vi "AnaliseOffline.vi"() -> ()   [LabVIEW 2014, in "Aquisicao de Dados.lvlib"]
uses:
  Aquisicao de Dados.lvlib
panel:
  in  "Amostras de Gravação":i32=100
  out "Waveform Graph":waveform(dbl)[](graph)
  in  "Método de Entrada":T1(ring)
  in  "Amostras por Iteração":i32=2000
  in  "Error In":errorcluster
  out "Error Out":errorcluster
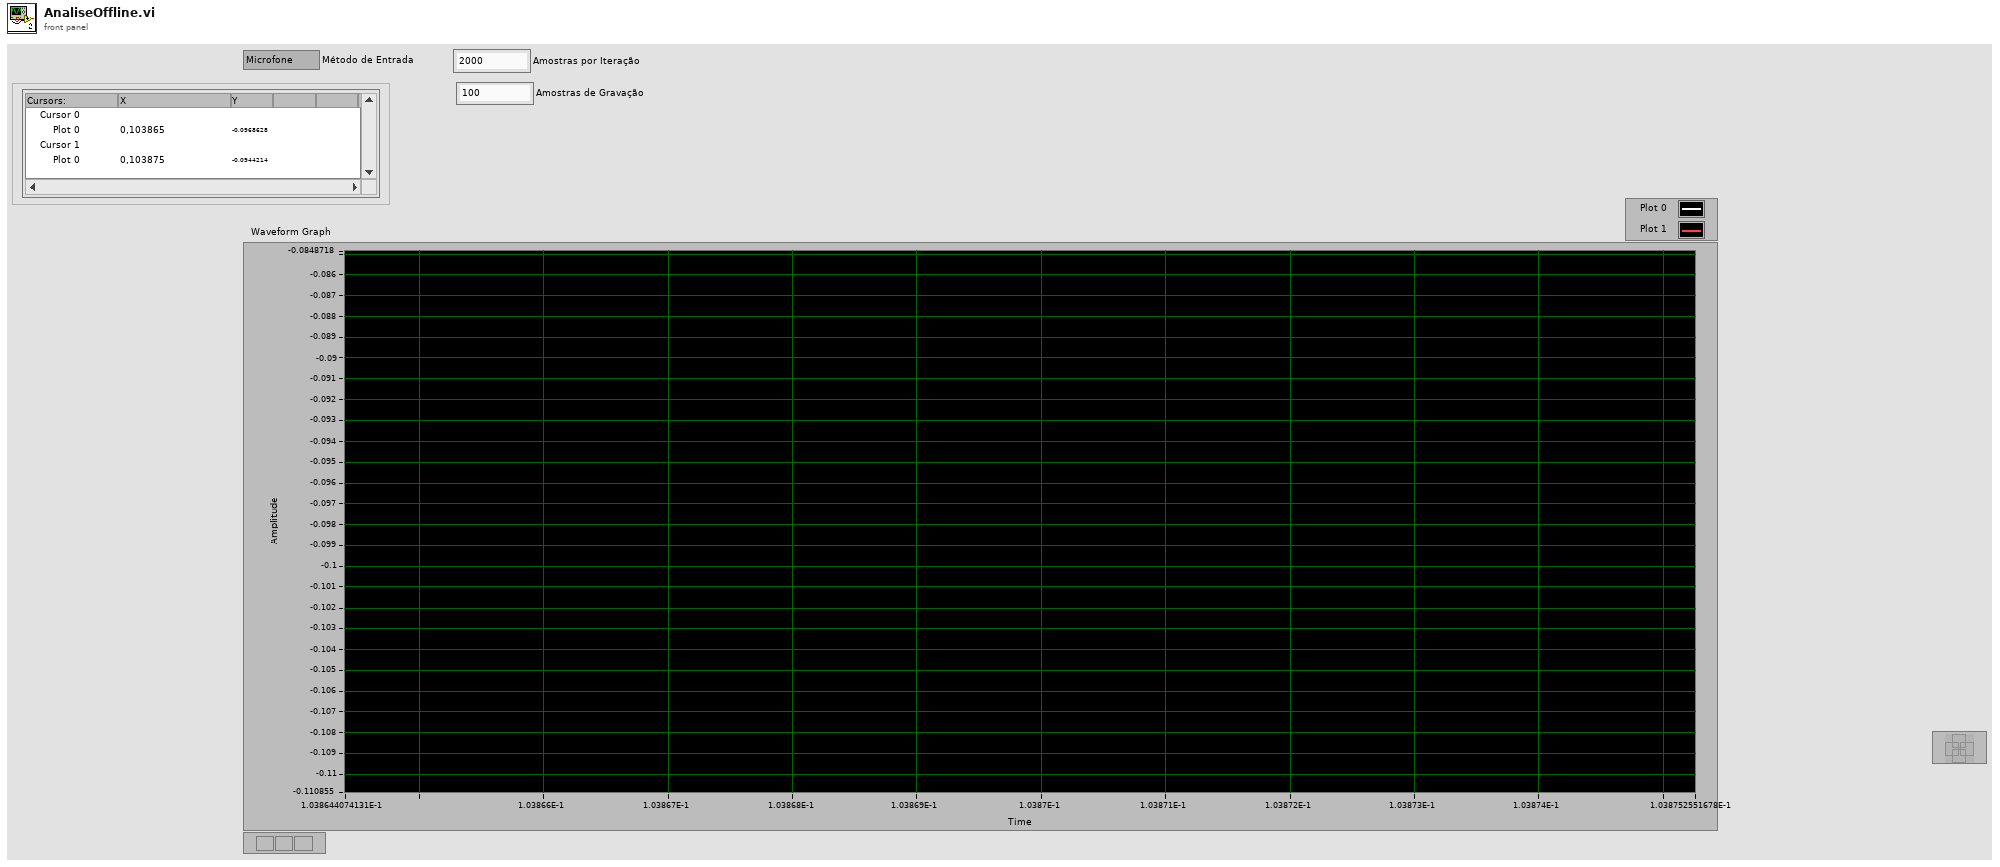
[diagram p1: front panel]
types:
  T1 = enum16{"Microfone", "Arduino", "LTSpice", "Arquivo WAV"}
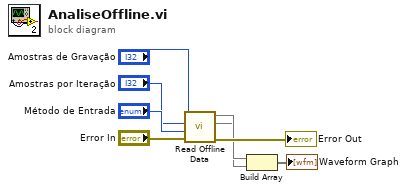
[diagram p0: block diagram]
diagram:
  n1 = call "Read Offline Data.vi"("Error In"="Error In", 9:"Método de Entrada", 10:"Amostras por Iteração", 11:"Amostras de Gravação") -> ("Error Out"=→"Error Out":errorcluster, 2:w2, 3:w3)  [unwired: 5 in]
  n2 = Build Array(w3, w2) -> (→"Waveform Graph":void[])
